vi "MockAccel.vi"(11 "MockAccelSettings":T1={"BufferUpdateFIFO"="MockAccelVoltageFIFO"}) -> ()   [LabVIEW 2016, in "FPGAMockAccel.lvlib"]
uses:
  FPGAMockAccel.lvlib
  DataTypes/MockAccelSettings.ctl
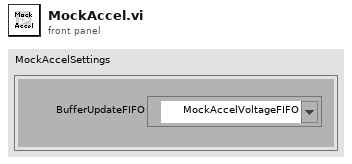
[diagram p1: front panel]
types:
  T1 = typedef "FPGAMockAccel.lvlib/MockAccelSettings.ctl" = cluster{"BufferUpdateFIFO":refnum<k21>}
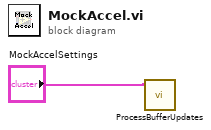
[diagram p0: block diagram]
diagram:
  n1 = call "ProcessBufferUpdates.vi"("MockAccelSettings"="MockAccelSettings") -> ()  [unwired: 11 in]
